vi "DWF PS Read Output.vi"(0 "Instrument Handle In":u32, 5 "Channel":string, 11 "Error In":errorcluster caption="Error In (no error)") -> (4 "Instrument Handle Out":u32, 6 "Actual Voltage Level":dbl, 8 "Actual Current Level":dbl, 10 "State":i32(ring) items=["Constant Current", "Constant Voltage"], 15 "Error Out":errorcluster)   [LabVIEW 2015, in "DigilentWF.lvlib"]
doc: "Reads the voltage and current levels of the specified channel."
uses:
  <vilib>/DigilentWF/DigilentWF.lvlib
  dwf.dll
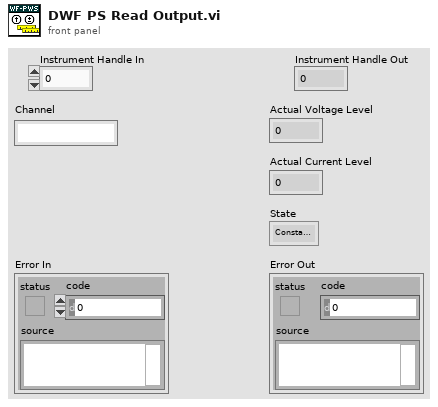
[diagram p1: front panel]
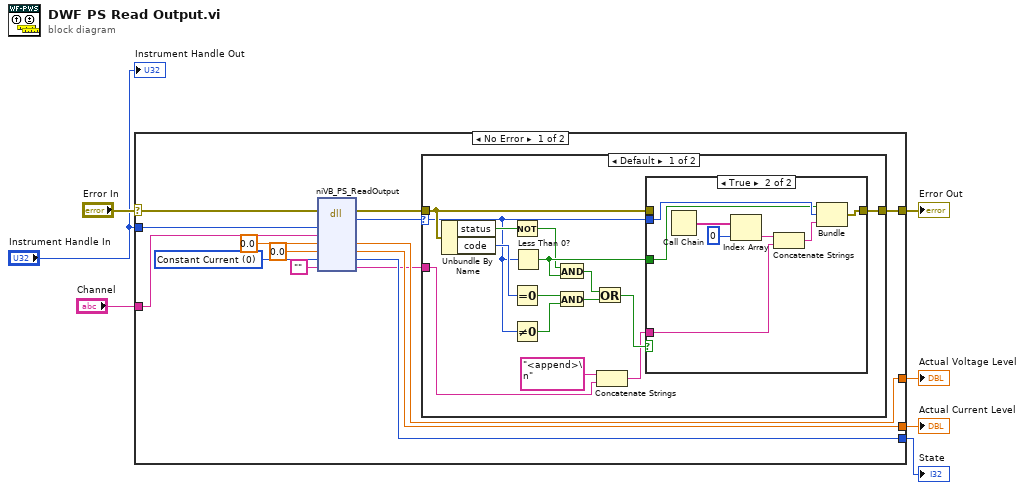
[diagram p0: block diagram]
diagram:
  n1 = case "outter_case" shown="No Error" "Error In" {
    selector: "Error In" -> [w20 w47]
    tunnel: [w21 w47] -> w6
    tunnel: "Instrument Handle In" -> [w17 _]
    tunnel: "Channel" -> [w16 _]
    tunnel: [w12 _] -> w3
    tunnel: [w11 _] -> w2
    tunnel: [w10 _] -> w1
    frame No Error {
      w15 = 0 items=["Constant Current", "Constant Voltage"] ("State")
      n2 = dll-call lib="dwf.*" fn="niVB_PS_ReadOutput"(error in=w20, "instrumentHandle"=w17, "channel"=w16, "actualVoltageLevel"=0.0 ("Actual Voltage Level"), "actualCurrentLevel"=0.0 ("Actual Current Level"), "state"=w15, "szError"="") -> (error out=w19:errorcluster, "return type"=w18:i32, "actualVoltageLevel"=w12:dbl, "actualCurrentLevel"=w11:dbl, "state"=w10:u32, "szError"=w8:string)  [unwired: 4 in, 1 out]
      n3 = case "inner_case" shown="Default" w18 {
        selector: w18 -> [w26 _]
        tunnel: w19 -> [w27 w46]
        tunnel: [w23 w46] -> w21
        tunnel: w8 -> [w22 _]
        frame Default {
          n4 = Unbundle By Name(w27) -> ("status"=w31:bool, "code"=w35:i32)
          n5 = Not(x=w31) -> (.not. x?=w34:bool)
          n6 = Equal To 0?(x=w35) -> (x = 0?=w30:bool)
          n7 = Not Equal To 0?(x=w26) -> (x != 0?=w33:bool)
          n8 = Less Than 0?(x=w26) -> (x < 0?=w36:bool)
          n9 = And(x=w34, y=w36) -> (x .and. y?=w32:bool)
          n10 = And(x=w30, y=w33) -> (x .and. y?=w29:bool)
          n11 = Or(x=w32, y=w29) -> (x .or. y?=w28:bool)
          n12 = Concatenate Strings("<append>\n" ("string"), w22) -> (w25:string)
          n13 = case shown="True" w28 {
            tunnel: [w37 w44] -> w23
            tunnel: w26 -> [_ w43]
            tunnel: w36 -> [_ w42]
            tunnel: w27 -> [w37 _]
            tunnel: w25 -> [_ w38]
            frame False {
            }
            frame True {
              n14 = Call Chain() -> (call chain=w41:string[])
              n15 = Index Array(array=w41, index=0) -> (element=w40:string)
              n16 = Concatenate Strings(w40, w38) -> (w45:string)
              n17 = Bundle(w42, "return type"=w43, w45) -> (w44:cluster{bool, "return type":i32, string})  [unwired: 1 out]
            }
          }
        }
        frame 0 {
        }
      }
    }
    frame Error {
    }
  }
  "Error Out" <- w6
  "Actual Voltage Level" <- w3
  "Actual Current Level" <- w2
  "State" <- w1
  "Instrument Handle Out" <- "Instrument Handle In"
